vi "File updated.vi"(8 "error in (no error)":errorcluster, 10 "File Path Control":path, 11 "MagLabGraph in":refnum<class "XY Plot.lvclass">) -> (0 "error out":errorcluster, 3 "MagLabGraph out":refnum<class "XY Plot.lvclass">)   [LabVIEW 2018, in "XY Plot.lvclass"]
uses:
  XY Plot.lvclass
  XY Plot.lvclass/XY Plot.ctl
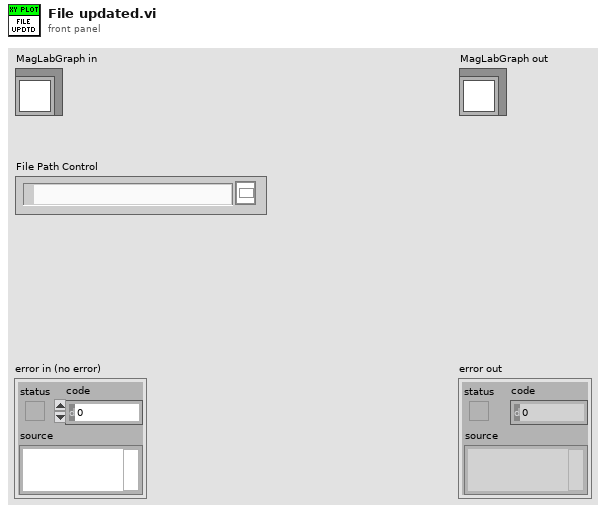
[diagram p1: front panel]
types:
  T1 = cluster{"File Path Control":path, "Group":string, "Channel":string, "Abbreviated":string}[]
  T2 = cluster{"File Path Control":path, "Group":string, "Channel":string, "Abbreviated":string}
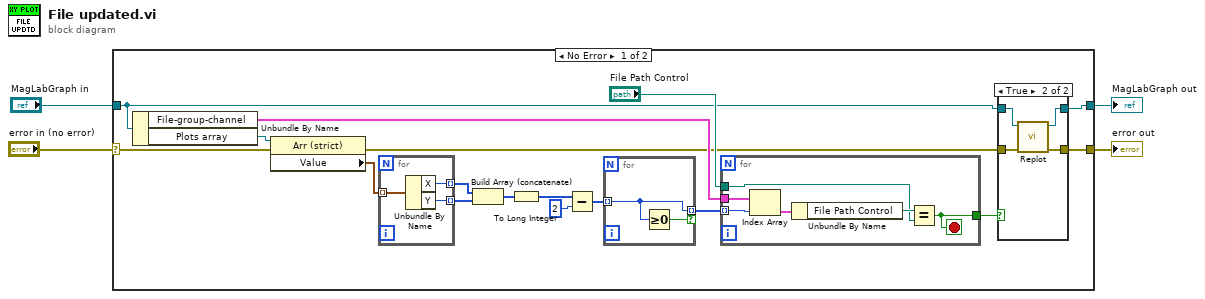
[diagram p0: block diagram]
diagram:
  n1 = case shown="No Error" "error in (no error)" {
    selector: "error in (no error)" -> [w14 w40]
    tunnel: [w6 w40] -> w3
    tunnel: [w8 w39] -> w1
    tunnel: "MagLabGraph in" -> [w15 w39]
    frame No Error {
      n2 = Unbundle By Name(w15) -> ("File-group-channel"=w17:T1, "Plots array"=w21:refnum<vi>)
      n3 = property class="Arr (strict)"(reference=w21, error in=w14) -> (error out=w7:errorcluster, "Value"=w20:cluster{"X":u16, "Y":u16}[])  [unwired: 1 out]
      n4 = for {
        tunnel: w20 -> [w38] mode=indexing
        tunnel: [w37] -> w19 mode=indexing
        tunnel: [w36] -> w18 mode=indexing
        n5 = Unbundle By Name(w38) -> ("X"=w37:u16, "Y"=w36:u16)
      }
      n6 = Build Array (concatenate)(w19, w18) -> (w13:u16[])
      n7 = To Long Integer(number=w13) -> (32bit integer=w11:i32[])
      n8 = Subtract(x=w11, y=2) -> (x-y=w10:i32[])
      n9 = for {
        tunnel: w10 -> [w29] mode=indexing
        tunnel: [w29] -> w9 mode=indexing if=w28
        n10 = Greater Or Equal To 0?(x=w29) -> (x >= 0?=w28:bool)
      }
      n11 = for {
        tunnel: w9 -> [w34] mode=indexing
        tunnel: w17 -> [w35]
        tunnel: "File Path Control" -> [w31]
        tunnel: [w30] -> w5
        stop <- w30 stop-if-true
        n12 = Index Array(array=w35, index=w34) -> (element=w33:T2)
        n13 = Unbundle By Name(w33) -> ("File Path Control"=w32:path)
        n14 = Equal?(x=w32, y=w31) -> (x = y?=w30:bool)
      }
      n15 = case shown="True" w5 {
        tunnel: w15 -> [w23 w27]
        tunnel: [w23 w26] -> w8
        tunnel: w7 -> [w22 w25]
        tunnel: [w22 w24] -> w6
        frame False {
        }
        frame True {
          n16 = call-dynamic "Replot.vi"("error in (no error)"=w25, "Plot in"=w27) -> ("error out"=w24:errorcluster, "Plot out"=w26:refnum<class "XY Plot.lvclass">)  [unwired: 8 in]
        }
      }
    }
    frame Error {
    }
  }
  "error out" <- w3
  "MagLabGraph out" <- w1
